vi "ReadData.vi"(8 "error in (no error)":errorcluster, 11 "RFSoC Driver in":refnum<class "RFSoC Driver.lvclass">) -> (0 "error out":errorcluster, 2 "Data out":i16[][](array[numeric]), 3 "RFSoC Driver out":refnum<class "RFSoC Driver.lvclass">)   [LabVIEW 2019, in "RFSoC Driver.lvclass"]
uses:
  RFSoC Driver.lvclass
  C:/GitHub/NHMFL_Core/Libraries/Instruments/RFSoC/2019/GitHub/NHMFL_Core/Libraries/Instruments/Pulse Driver/Pulse Driver.lvclass
  Pulse Driver/Pulse Driver.lvclass/Pulse Driver.ctl
  RFSoC Driver.lvclass/RFSoC Driver.ctl
  Pulse Driver/Read Samples per read.vi
  Read Mixer.vi
panel:
  out "Extra data out":string
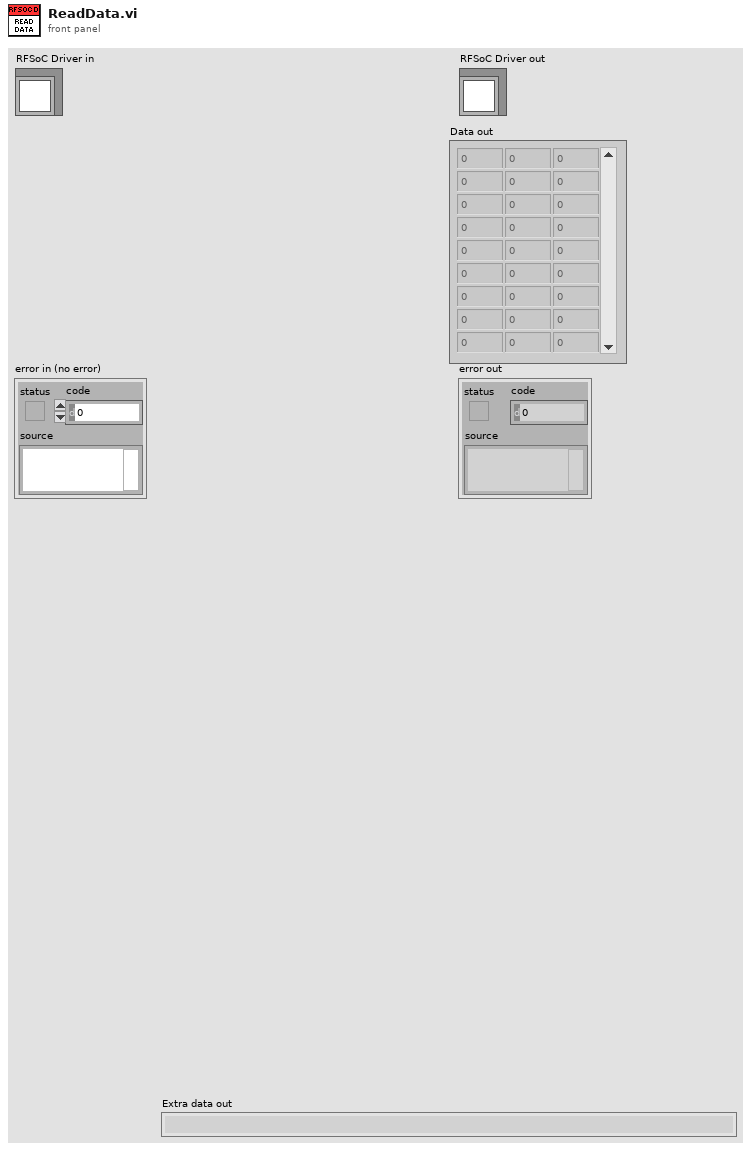
[diagram p1: front panel]
types:
  T1 = enum16{"big-endian, network order", "native, host order", "little-endian"}
  T2 = enum16{"Standard", "Buffered", "CRLF", "Immediate"}
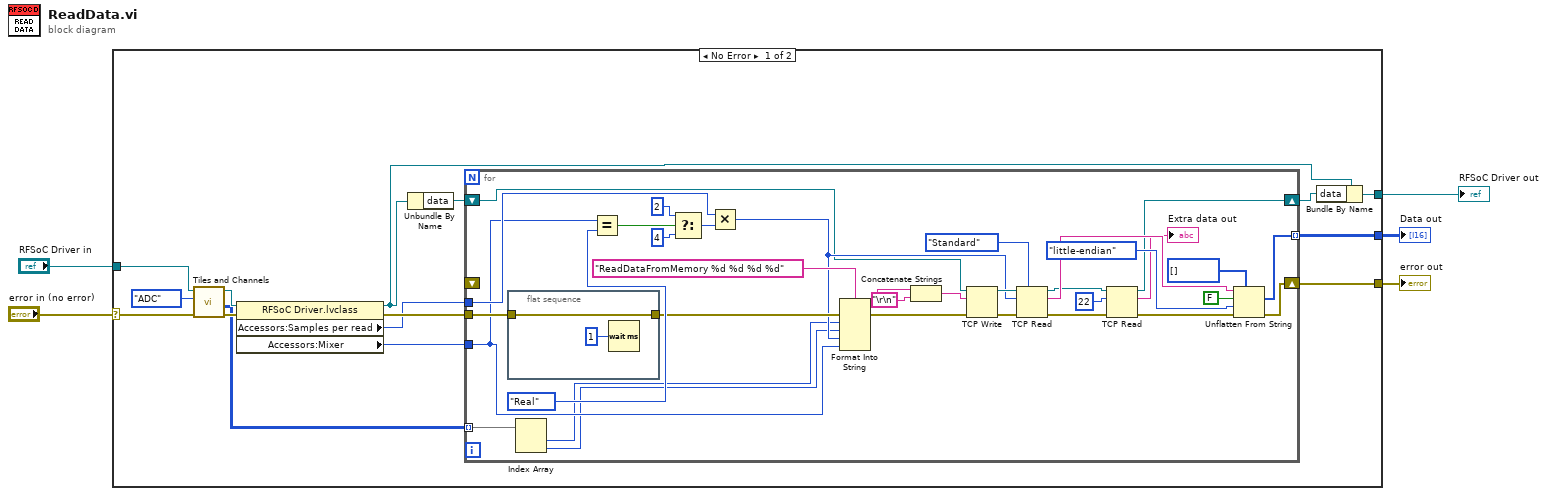
[diagram p0: block diagram]
diagram:
  n1 = case shown="No Error" "error in (no error)" {
    selector: "error in (no error)" -> [w9 w58]
    tunnel: [w20 w58] -> w4
    tunnel: [w12 w57] -> w2
    tunnel: "RFSoC Driver in" -> [w11 w57]
    tunnel: [w16 _] -> w1
    frame No Error {
      n2 = call-dynamic "Tiles and Channels.vi"("error in (no error)"=w9, "Type"=enum16{"ADC", "DAC"}."ADC", "RFSoC Driver in"=w11) -> ("error out"=w7:errorcluster, "Tiles and converters out"=w6:i32[][], "RFSoC Driver out"=w10:refnum<class "RFSoC Driver.lvclass">)  [unwired: 5 in, 1 out]
      n3 = property class="RFSoC Driver.lvclass"(reference=w10, error in=w7) -> (reference out=w15:refnum<class "RFSoC Driver.lvclass">, error out=w19:errorcluster, "Accessors:Samples per read"=w18:i32, "Accessors:Mixer"=w17:enum16{"Real", "I/Q"})
      n4 = Unbundle By Name(w15) -> ("data"=w14:refnum<k5>)
      n5 = for {
        shift-right: [w31] -> w20
        shift-left: _ -> [_]
        tunnel: [w30] -> w16 mode=indexing
        tunnel: w19 -> [w28]
        tunnel: w18 -> [w27]
        tunnel: w17 -> [w26]
        tunnel: w6 -> [w23] mode=indexing
        shift-right: [w24] -> w13
        shift-left: w14 -> [w25]
        n6 = flat-sequence {
          tunnel: [w55] -> w33
          tunnel: w28 -> [w55]
          frame #0 {
            n7 = Wait (ms)(milliseconds to wait=u32 1) -> ()  [unwired: 1 out]
          }
        }
        n8 = Index Array(array=w23) -> (element #1=w22:i32, element #2=w21:i32)  [unwired: 2 in]
        n9 = Equal?(x=w26, y=enum16{"Real", "I/Q"}."Real" ("Mixer")) -> (x = y?=w39:bool)
        n10 = Select(t=2 ("Binary sample width"), s=w39, f=4 ("Binary sample width")) -> (s? t:f=w35:i32)
        n11 = Multiply(x=w27, y=w35) -> (x*y=w29:i32)
        n12 = Format Into String(format string="ReadDataFromMemory %d %d %d %d", error in=w33, w22, w21, w29, w26) -> (resulting string=w34:string, error out=w32:errorcluster)  [unwired: 1 in]
        n13 = Concatenate Strings(w34, "\r\n") -> (w53:string)
        n14 = TCP Write(connection ID=w25, data in=w53, error in (no error)=w32) -> (connection ID out=w51:refnum<k5>, error out=w52:errorcluster)  [unwired: 1 in, 1 out]
        n15 = TCP Read(connection ID=w51, bytes to read=w29, error in (no error)=w52, 7:T2."Standard" ("mode (standard)")) -> (connection ID out=w43:refnum<k5>, data out=w49:string, error out=w45:errorcluster)  [unwired: 1 in]
        n16 = TCP Read(connection ID=w43, bytes to read=22, error in (no error)=w45) -> (connection ID out=w24:refnum<k5>, data out=→"Extra data out":string, error out=w44:errorcluster)  [unwired: 2 in]
        n17 = Unflatten From String(type=i16[] [], binary string=w49, data includes array or string size? (T)=FALSE, byte order (0:big-endian, network order)=T1."little-endian", error in (no error)=w44) -> (value=w30:i16[], error out=w31:errorcluster)  [unwired: 1 out]
      }
      n18 = Bundle By Name(cluster=w15, "data"=w13) -> (w12:refnum<class "RFSoC Driver.lvclass">)
    }
    frame Error {
    }
  }
  "error out" <- w4
  "RFSoC Driver out" <- w2
  "Data out" <- w1
